vi "Load image from dedicated folder.vi"(8 "error in (no error)":errorcluster, 10 "name or relative path":string, 11 "2D Picture ctrl ref":refnum<vi>) -> (0 "error out":errorcluster)   [LabVIEW 2020]
uses:
  Typedefs/Which path.ctl
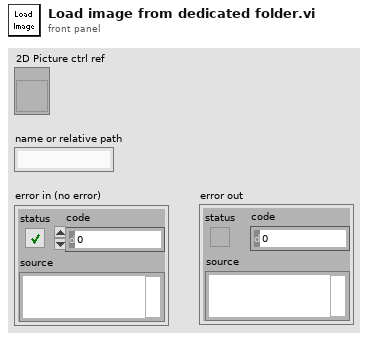
[diagram p1: front panel]
types:
  T1 = typedef "Which path.ctl" = enum16{"Configuration Files", "Calibration Files", "Images", "Setup.ini", "Loaded User profile.ini", "User's-Previous session.ini", "New user profile.ini", "Selected User profile.ini", "User profiles folder", "Power meter scaling.txt", "FOV Cal.ini", "Calibration.ini"}
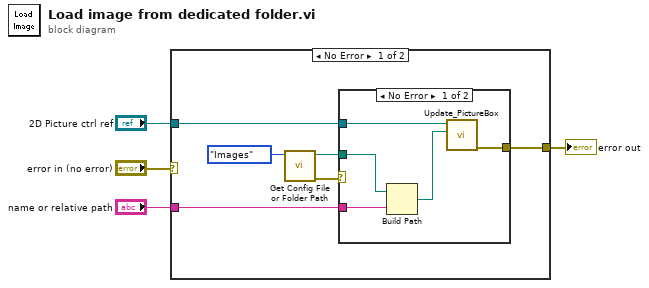
[diagram p0: block diagram]
diagram:
  n1 = case shown="No Error" "error in (no error)" {
    selector: "error in (no error)" -> [_ w17]
    tunnel: "2D Picture ctrl ref" -> [w10 _]
    tunnel: "name or relative path" -> [w8 _]
    tunnel: [w6 w17] -> w3
    frame No Error {
      n2 = call "Get Config File or Folder Path.vi"("Which file or folder?"=Which_path."Images") -> ("Error Out"=w5:errorcluster, "File Path"=w7:path)  [unwired: 8 in, 1 out]
      n3 = case shown="No Error" w5 {
        selector: w5 -> [_ w16]
        tunnel: w10 -> [w15 _]
        tunnel: w8 -> [w14 _]
        tunnel: w7 -> [w13 _]
        tunnel: [w11 w16] -> w6
        frame No Error {
          n4 = Build Path(base path=w13, name or relative path=w14) -> (appended path=w12:path)
          n5 = call <userlib>:"Update_PictureBox.vi"("Picture Path"=w12, "Picture Box in"=w15) -> ("error out"=w11:errorcluster)  [unwired: 5 in, 4 out]
        }
        frame Error {
        }
      }
    }
    frame Error {
    }
  }
  "error out" <- w3
